vi "del 0 item.vi"(9 "Array in":dbl[](array[numeric]), 10 "Y":dbl[](array[numeric]), 11 "x in":dbl[](array[numeric])) -> (2 "Array out":dbl[](array[numeric]), 3 "x out":dbl[](array[numeric]))   [LabVIEW 2019]
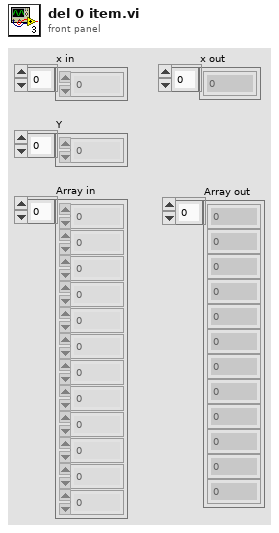
[diagram p1: front panel]
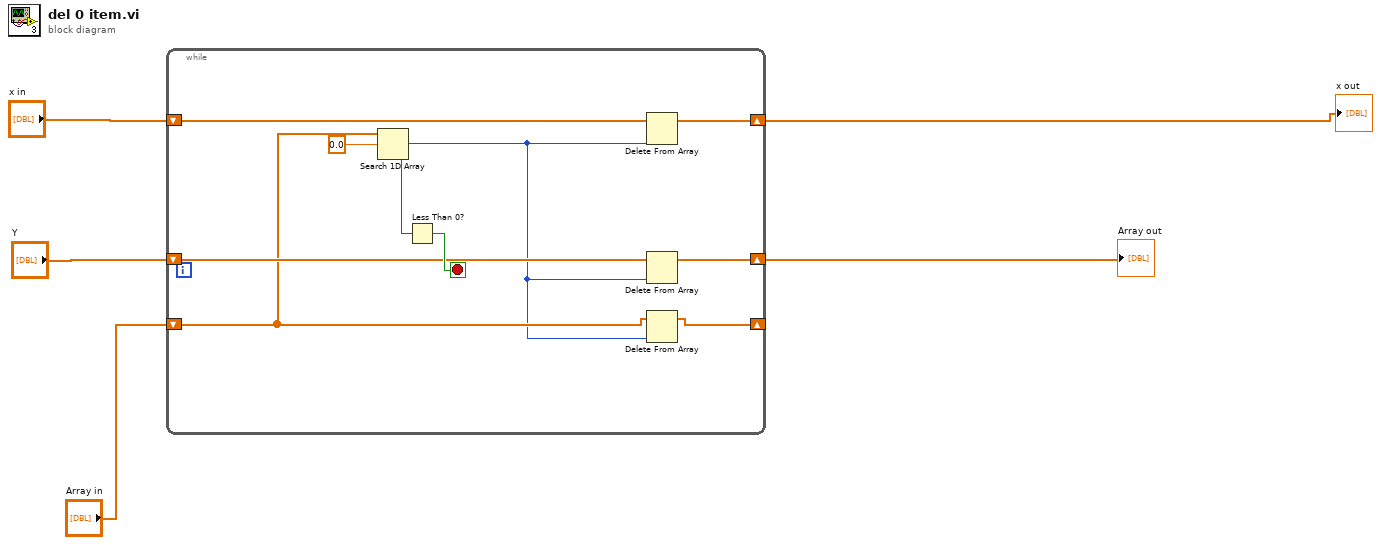
[diagram p0: block diagram]
diagram:
  n1 = while {
    shift-right: [w6] -> _
    shift-left: "Array in" -> [w8]
    shift-right: [w10] -> w2
    shift-left: "Y" -> [w12]
    shift-right: [w9] -> w1
    shift-left: "x in" -> [w11]
    stop <- w13 stop-if-true
    n2 = Search 1D Array(1D array=w8, element=0.0) -> (index of element=w7:i32)  [unwired: 1 in]
    n3 = Less Than 0?(x=w7) -> (x < 0?=w13:bool)
    n4 = Delete From Array(array=w11, index=w7) -> (array with subset deleted=w9:dbl[])  [unwired: 1 in, 1 out]
    n5 = Delete From Array "Delete From Array"(array=w12, index=w7) -> (array with subset deleted=w10:dbl[])  [unwired: 1 in, 1 out]
    n6 = Delete From Array(array=w8, index=w7) -> (array with subset deleted=w6:dbl[])  [unwired: 1 in, 1 out]
  }
  "Array out" <- w2
  "x out" <- w1
